vi "Get Xbox One Controller State.vi"(8 "error in (no error)":errorcluster, 11 "Operator in":refnum<class "Operator.lvclass">) -> (0 "error out":errorcluster, 2 "Xbox One Controller":T1 {"Right Joystick"."Right" min=-1.0 max=1.0 step=0.1 scale=-1.0..1.0; "Right Joystick"."Forward" min=-1.0 max=1.0 step=0.1 scale=-1.0..1.0; "Left Joystick"."Right" min=-1.0 max=1.0 step=0.1 scale=-1.0..1.0; "Left Joystick"."Forward" min=-1.0 max=1.0 step=0.1 scale=-1.0..1.0}, 3 "Operator out":refnum<class "Operator.lvclass">)   [LabVIEW 2014, in "Operator.lvlib" / "Operator.lvclass"]
uses:
  Operator.lvclass
  Xbox One Controller/Xbox One Controller State.ctl
  Xbox One Controller/Joystick.ctl
  Xbox One Controller/Xbox One Controller.lvlib
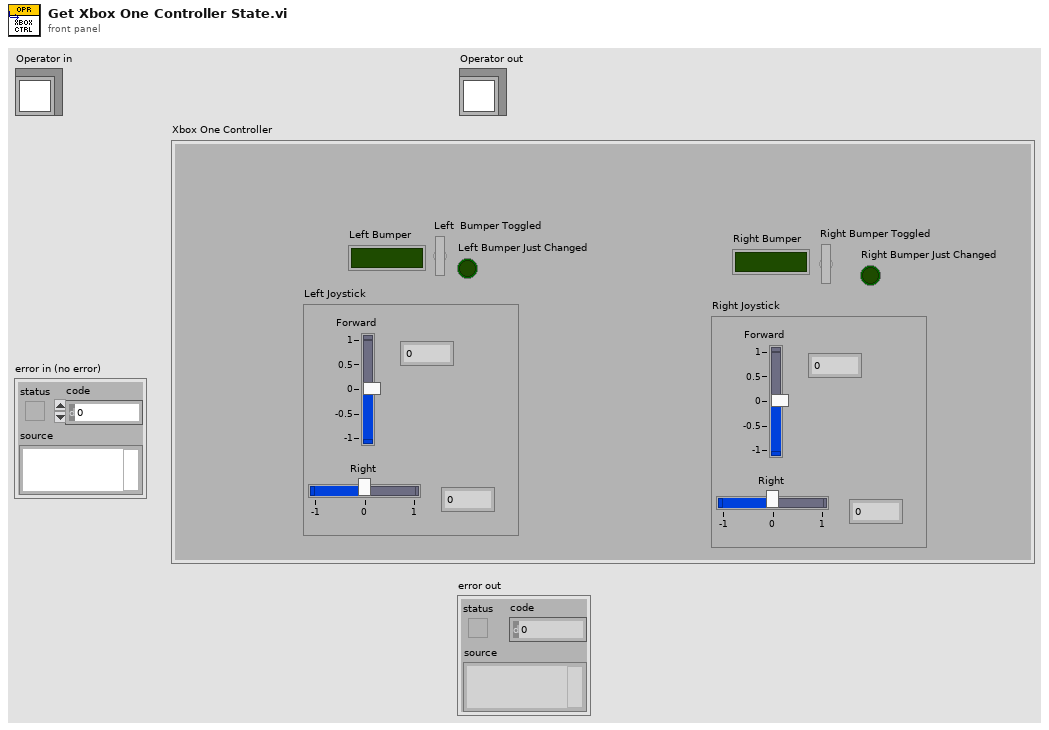
[diagram p1: front panel]
types:
  T1 = typedef "Xbox One Controller.lvlib/Xbox One Controller State.ctl" = cluster{"Left Joystick":T2, "Right Joystick":T2, "Right Bumper":bool, "Left Bumper":bool, "Left  Bumper Toggled":bool, "Right Bumper Toggled":bool, "Left Bumper Just Changed":bool, "Right Bumper Just Changed":bool}
  T2 = typedef "Xbox One Controller.lvlib/Joystick.ctl" = cluster{"Forward":dbl, "Right":dbl}
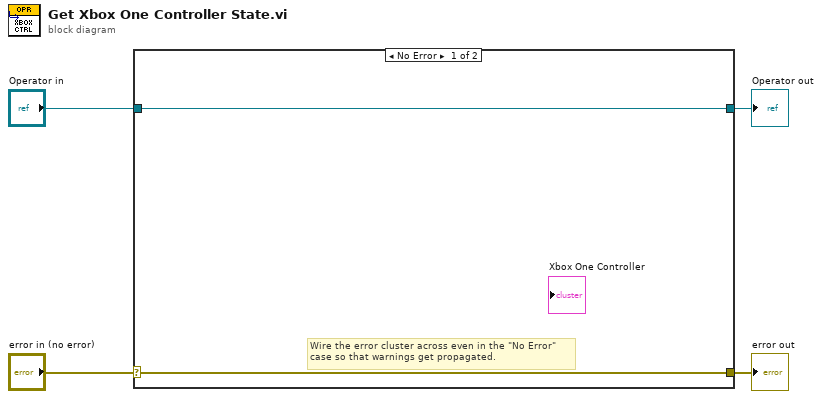
[diagram p0: block diagram]
diagram:
  n1 = case shown="No Error" "error in (no error)" {
    selector: "error in (no error)" -> [w5 w8]
    tunnel: [w5 w8] -> w3
    tunnel: [w6 w7] -> w1
    tunnel: "Operator in" -> [w6 w7]
    frame No Error {
      # "Wire the error cluster across even in the \"No Error\"\ncase so that warnings get propagated."
    }
    frame Error {
    }
  }
  "error out" <- w3
  "Operator out" <- w1
